vi "Activity_6.vi"() -> ()   [LabVIEW 2015]
panel:
  out "replaced substring":string="C:\\Users\\leser\\Dropbox\\"
  out "result string":string="Hello: Equipo9\\Activity_5.viLuis Esteban SerranoInstrumentacionVirtual"
  in  "length (len. of substring)":i32=23
  in  "offset (0)":i32
  in  "substring (\"\")":string="Hello: "
  in  "length (rest)":i32=86
  out "substring":string="C:\\Users\\leser\\Dropbox\\Equipo9\\Activity_5.viLuis Esteban SerranoInstrumentacionVirtual"
  out "concatenated string":string="C:\\Users\\leser\\Dropbox\\Equipo9\\Activity_5.viLuis Esteban SerranoInstrumentacionVirtual"
  out "length":i32=44
  out "String":string="C:\\Users\\leser\\Dropbox\\Equipo9\\Activity_5.vi"
  in  "Path":path=path "C:/Users/leser/Dropbox/Equipo9/Activity_5.vi"
  # "Modificacion de Cadenas"
  # "Serrano Bermúdez Luis Esteban\nFecha de Entrega 17/02/2019"
  # "Descripcion: Esta aplicacion usa 2 cadenas constantes iniciales para\nconcatenarlas a un Path que será convertido a cadena.\nAdicionalmente se puede usar la casilla de \"suubstring\" para incluir \nuna subcadena en un lugar elegido de la cadena principal, para ello\nse elige la posicion por medio del offset y el tamaño de la cadena\nque se va a reemplazar"
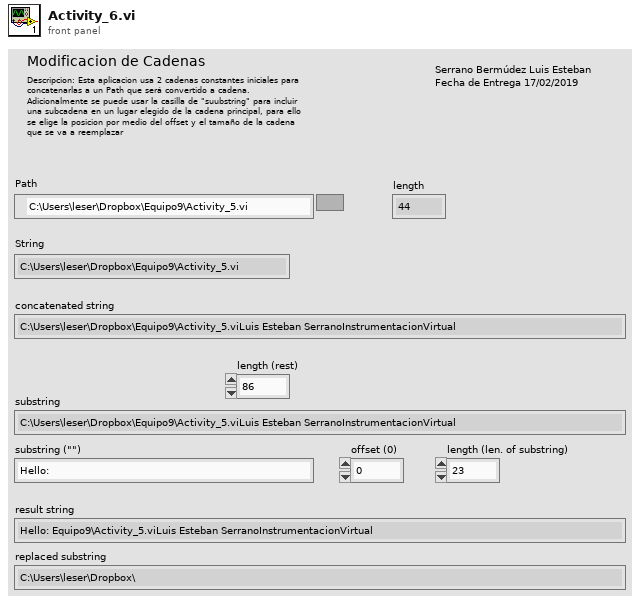
[diagram p1: front panel]
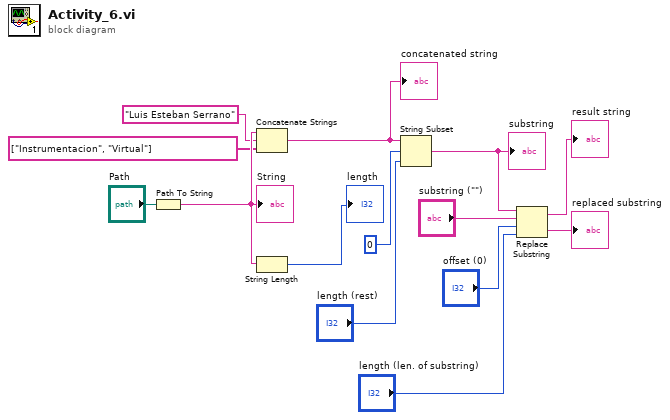
[diagram p0: block diagram]
diagram:
  n1 = Path To String(path="Path") -> (string=w12:string)
  "String" <- w12
  n2 = Concatenate Strings "Concatenate Strings"(w12, "Luis Esteban Serrano", string[] ["Instrumentacion", "Virtual"]) -> (w9:string)
  "concatenated string" <- w9
  n3 = String Length(string=w12) -> (length=→"length":i32)
  n4 = String Subset(string=w9, offset (0)=0, length (rest)="length (rest)") -> (substring=w7:string)
  "substring" <- w7
  n5 = Replace Substring(2:"length (len. of substring)", 3:"offset (0)", 4:"substring (\"\")", 5:w7) -> (0:→"replaced substring":string, 1:→"result string":string)
